vi "SumNoiseFloor.vi"(8 "df":dbl, 9 "Width [bins]":dbl[](array[numeric]), 10 "frequencies to remove [Hz]":dbl[](array[numeric]), 11 "Spectrum_dBm":dbl[](array[numeric])) -> (3 "Numeric":dbl)   [LabVIEW 2018]
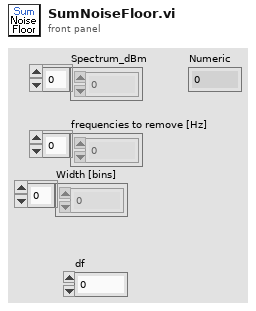
[diagram p1: front panel]
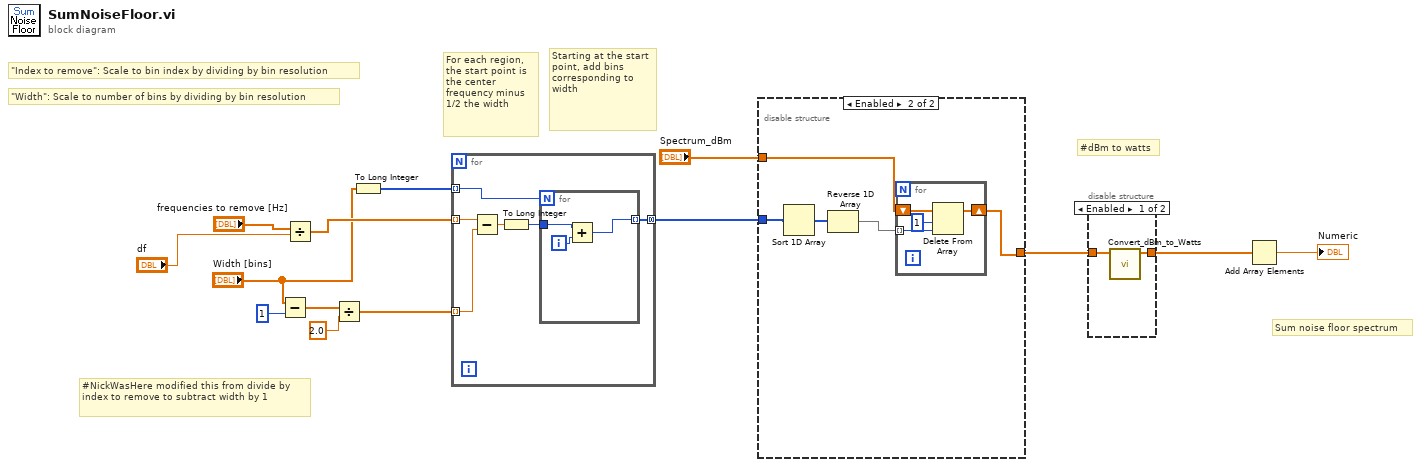
[diagram p0: block diagram]
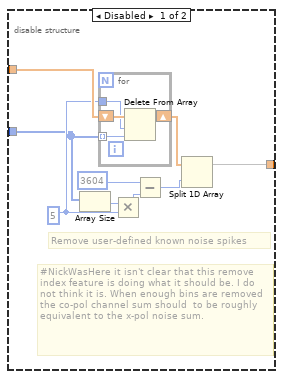
[diagram p2: hidden frame]
diagram:
  # "#NickWasHere modified this from divide by index to remove to subtract width by 1"
  # "Starting at the start point, add bins corresponding to width"
  # "For each region, the start point is the center frequency minus 1/2 the width"
  # "\"Width\": Scale to number of bins by dividing by bin resolution"
  # "\"Index to remove\": Scale to bin index by dividing by bin resolution"
  # "#dBm to watts"
  # "Sum noise floor spectrum"
  n1 = Subtract(x="Width [bins]", y=1) -> (x-y=w8:dbl[])
  n2 = Divide(x="frequencies to remove [Hz]", y="df") -> (x/y=w6:dbl[])
  n3 = Divide(x=w8, y=2.0) -> (x/y=w4:dbl[])
  n4 = To Long Integer(number="Width [bins]") -> (32bit integer=w3:i32[])
  n5 = for {
    tunnel: w6 -> [w20] mode=indexing
    tunnel: [w16] -> w5 mode=concatenating
    tunnel: w4 -> [w19] mode=indexing
    tunnel: w3 -> [w17] mode=indexing
    n6 = Subtract(x=w20, y=w19) -> (x-y=w18:dbl)
    n7 = To Long Integer(number=w18) -> (32bit integer=w15:i32)
    n8 = for {
      N: w17 -> [_]
      tunnel: w15 -> [w23]
      tunnel: [w21] -> w16 mode=indexing
      i -> [w22]
      n9 = Add(x=w23, y=w22) -> (x+y=w21:i32)
    }
  }
  n10 = disable-structure shown="Enabled" {
    disable-tunnel: "Spectrum_dBm" -> [w32 w39]
    disable-tunnel: [w25 w37] -> w12
    disable-tunnel: w5 -> [w24 w41]
    frame Disabled {
      w28 = 5 ("#toRemove")
      # "#NickWasHere it isn't clear that this remove index feature is doing what it should be. I do not think it is. When enough bins are removed the co-pol channel sum should  to be roughly equivalent to the x-pol noise sum."
      # "Remove user-defined known noise spikes"
      n11 = Array Size(array=w24) -> (size(s)=w29:i32)
      n12 = for {
        tunnel: w28 -> [w34]
        tunnel: w24 -> [w33] mode=indexing
        shift-right: [w35] -> w31
        shift-left: w32 -> [w36]
        n13 = Delete From Array(array=w36, length=w34, index=w33) -> (array with subset deleted=w35:dbl[])  [unwired: 1 out]
      }
      n14 = Multiply(x=w29, y=w28) -> (x*y=w27:i32)
      n15 = Subtract(x=3604 ("index"), y=w27) -> (x-y=w26:i32)
      n16 = Split 1D Array(array=w31, index=w26) -> (first subarray=w25:dbl[])  [unwired: 1 out]
    }
    frame Enabled {
      n17 = Sort 1D Array(array=w41) -> (sorted array=w40:i32[])
      n18 = Reverse 1D Array(array=w40) -> (reversed array=w38:i32[])
      n19 = for {
        shift-right: [w44] -> w37
        shift-left: w39 -> [w45]
        tunnel: w38 -> [w43] mode=indexing
        n20 = Delete From Array(array=w45, length=1, index=w43) -> (array with subset deleted=w44:dbl[])  [unwired: 1 out]
      }
    }
  }
  n21 = disable-structure shown="Enabled" {
    disable-tunnel: w12 -> [w47 w48]
    disable-tunnel: [w46 w48] -> w11
    frame Enabled {
      n22 = call "Convert_dBm_to_Watts.vi"("P(dBm)"=w47) -> ("P(n_watts)"=w46:dbl[])  [unwired: 10 in]
    }
    frame Disabled {
    }
  }
  n23 = Add Array Elements(numeric array=w11) -> (sum=→"Numeric":dbl)
